vi "Yokogawa.vi"(0 "V/A ?":enum16{"DC V", "DC A"}(ring), 1 "Bias":enum16{"Low", "High"}(ring), 2 "Delay [ms]":u32=500, 3 "Messzeit [ms]":u32=5000, 4 "B-Feld":dbl, 5 "error in (no error)":errorcluster, 6 "Startwert":dbl=-5.0 min=-5.0 max=5.0 step=1.0, 7 "Stepsize":dbl=1.0 min=0.0, 8 "Endwert":dbl=5.0 min=-5.0 max=5.0 step=1.0) -> (15 "Ausgabe-Cluster":T1 {"Timestamp" format="%#_6f"}, 19 "error out":errorcluster)   [LabVIEW 2009]
uses:
  Instance           2 16Saved   Yokogawa .vi
panel:
  out "Done":bool
  out "Data":bool
  out "UI":dbl=12.99010000000002
  out "Modus":string="F1SA"
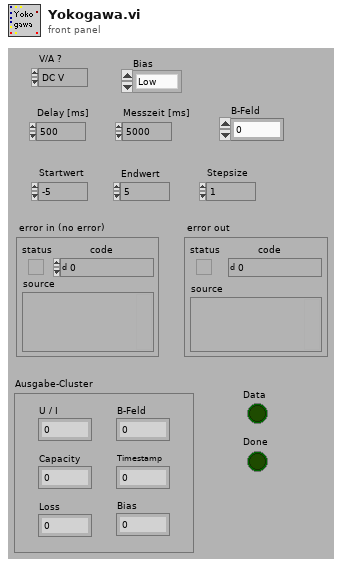
[diagram p1: front panel]
types:
  T1 = cluster{"U / I":dbl, "Capacity":dbl, "Loss":dbl, "B-Feld":dbl, "Timestamp":dbl, "Bias":u32}
  T2 = cluster{"UI":dbl, "capacitance":dbl, "loss":dbl, "B-Feld":dbl, dbl, "Bias":enum16{"Low", "High"}}
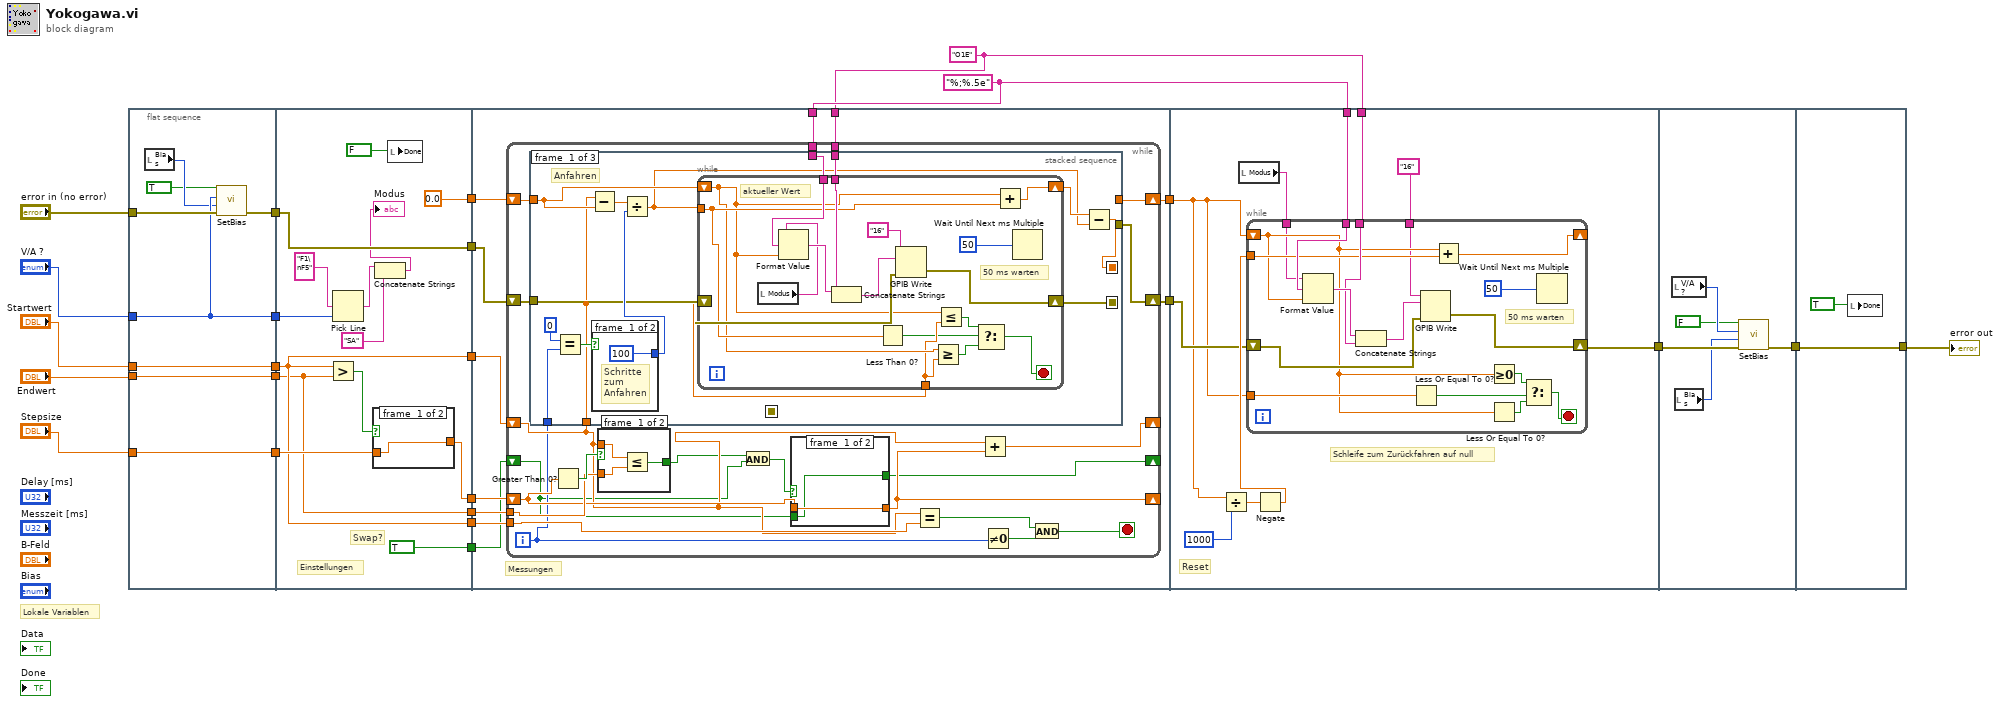
[diagram p0: block diagram]
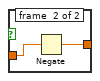
[diagram p2: hidden frame]
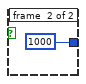
[diagram p3: hidden frame]
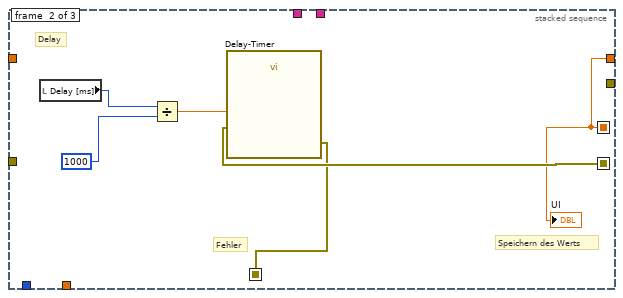
[diagram p4: hidden frame]
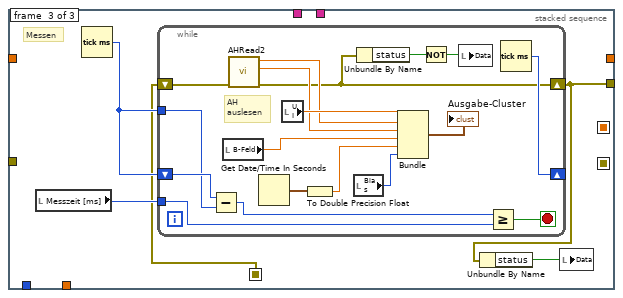
[diagram p5: hidden frame]
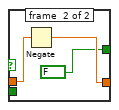
[diagram p6: hidden frame]
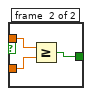
[diagram p7: hidden frame]
diagram:
  w9 = "O1E"
  w10 = "%;%.5e"
  # "Lokale Variablen"
  n1 = flat-sequence {
    tunnel: "Stepsize" -> [w30]
    tunnel: "Endwert" -> [w31]
    tunnel: "Startwert" -> [w32]
    tunnel: "V/A ?" -> [w27]
    tunnel: "error in (no error)" -> [w29]
    tunnel: [w28] -> w7
    tunnel: [w27] -> w6
    tunnel: [w32] -> w5
    tunnel: [w31] -> w4
    tunnel: [w30] -> w3
    tunnel: [w41] -> w19
    tunnel: [w42] -> w18
    tunnel: [w41] -> w17
    tunnel: [w40] -> w16
    tunnel: [0.0] -> w15
    tunnel: [w35] -> w14
    tunnel: [TRUE] -> w13
    tunnel: w7 -> [w35]
    tunnel: w6 -> [w45]
    tunnel: w5 -> [w41]
    tunnel: w4 -> [w40]
    tunnel: w3 -> [w43]
    tunnel: w19 -> [w60]
    tunnel: w18 -> [w58]
    tunnel: w17 -> [w59]
    tunnel: w16 -> [w57]
    tunnel: w15 -> [w56]
    tunnel: w10 -> [w55]
    tunnel: w9 -> [w54]
    tunnel: w14 -> [w53]
    tunnel: w13 -> [w51]
    tunnel: [w52] -> w12
    tunnel: [w50] -> w11
    tunnel: w12 -> [w159]
    tunnel: w11 -> [w157]
    tunnel: w10 -> [w161]
    tunnel: w9 -> [w160]
    tunnel: [w158] -> w2
    tunnel: w2 -> [w185]
    tunnel: [w186] -> w1
    tunnel: [w188] -> w8
    tunnel: w1 -> [w188]
    frame #0 {
      n2 = local read "Bias"() -> (w26:enum16{"Low", "High"})
      n3 = call "SetBias.vi"("error in (no error)"=w29, "Bias"=w26, "V/A ?"=w27, "On/Off"=TRUE) -> ("error out"=w28:errorcluster)  [unwired: 7 in]
    }
    frame #1 {
      # "Einstellungen"
      # "Swap?"
      n4 = Greater?(x=w41, y=w40) -> (0:w44:bool)
      n5 = Pick Line(multi-line string="F1\nF5", line index=w45) -> (output string=w38:string)  [unwired: 1 in]
      n6 = case shown="True" w44 {
        tunnel: w43 -> [w47 w49]
        tunnel: [w47 w48] -> w42
        frame #0 {
        }
        frame #1 {
          n7 = Negate(x=w49) -> (-x=w48:dbl)
        }
      }
      n8 = Concatenate Strings(w38, "SA") -> (→"Modus":string)
      n9 = local write "Done"(FALSE) -> ()
    }
    frame #2 {
      # "Messungen"
      n10 = while {
        shift-right: [w70] -> _
        shift-left: w60 -> [w72]
        tunnel: w59 -> [w81]
        shift-right: [w71] -> _
        shift-left: w58 -> [w78]
        tunnel: w57 -> [w79]
        shift-right: [w73] -> w50
        shift-left: w56 -> [w77]
        tunnel: w55 -> [w76]
        tunnel: w54 -> [w75]
        shift-right: [w69] -> w52
        shift-left: w53 -> [w74]
        shift-right: [w64] -> _
        shift-left: w51 -> [w62]
        i -> [w68]
        stop <- w65 stop-if-true
        n11 = stacked-sequence {
          seq-local: [w87 _ _] -> [_ w120 _]
          seq-local: [_ w119 _] -> [_ _ w123]
          seq-local: [w82 _ _] -> [_ w115 _]
          tunnel: w68 -> [w94 _ _]
          tunnel: w77 -> [w86 _ _]
          tunnel: w72 -> [w85 _ _]
          tunnel: w76 -> [w90 _ _]
          tunnel: w75 -> [w89 _ _]
          tunnel: w74 -> [w88 _ _]
          tunnel: [_ w115 _] -> w73
          tunnel: [_ _ w122] -> w69
          frame #0 {
            # "Anfahren"
            n12 = Equal?(x=0, y=w94) -> (x = y?=w95:bool)
            n13 = Subtract(x=w85, y=w86) -> (x-y=w92:dbl)
            n14 = case shown="True" w95 {
              tunnel: [100 1000] -> w91
              frame #0 {
                # "Schritte\nzum\nAnfahren"
              }
              frame #1 {
              }
            }
            n15 = Divide(x=w92, y=w91) -> (x/y=w83:dbl)
            n16 = while {
              shift-right: [w112] -> w84
              shift-left: w86 -> [w103]
              tunnel: w85 -> [w102]
              tunnel: w83 -> [w104]
              tunnel: w90 -> [w111]
              tunnel: w89 -> [w109]
              shift-right: [w106] -> w87
              shift-left: w88 -> [w107]
              stop <- w98 stop-if-true
              # "50 ms warten"
              # "aktueller Wert"
              n17 = local read "Modus"() -> (w96:string)
              n18 = Format Value(string ("")=w96, format string=w111, value (0)=w103) -> (output string=w110:string)
              n19 = Concatenate Strings(w110, w109) -> (w108:string)
              n20 = Less Than 0?(x=w104) -> (x < 0?=w101:bool)
              n21 = GPIB Write(0:"16", 1:w108, 3:w107) -> (6:w106:errorcluster)  [unwired: 2 in, 1 out]
              n22 = Greater Or Equal?(x=w103, y=w102) -> (x >= y?=w99:bool)
              n23 = Less Or Equal?(x=w103, y=w102) -> (x <= y?=w100:bool)
              n24 = Select(t=w100, s=w101, f=w99) -> (s? t:f=w98:bool)
              n25 = Add(x=w103, y=w104) -> (x+y=w112:dbl)
              n26 = Wait Until Next ms Multiple(millisecond multiple=50) -> ()  [unwired: 1 out]
            }
            n27 = Subtract(x=w84, y=w83) -> (x-y=w82:dbl)
          }
          frame #1 {
            # "Delay"
            # "Speichern des Werts"
            # "Fehler"
            n28 = local read "Delay [ms]"() -> (w116:u32)
            n29 = Divide(x=w116, y=u32 1000) -> (x/y=w117:dbl)
            n30 = call "Delay-Timer"("error in (no error)"=w120, "Delay Time (s)"=w117) -> ("error out"=w119:errorcluster)  [unwired: 9 in]
            "UI" <- w115
          }
          frame #2 {
            # "Messen"
            n31 = local read "Messzeit [ms]"() -> (w124:u32)
            n32 = Tick Count (ms)() -> (millisecond timer value=w125:u32)
            n33 = while {
              shift-right: [w143] -> _
              shift-left: w125 -> [w142]
              tunnel: w125 -> [w141]
              tunnel: w124 -> [w139]
              shift-right: [w127] -> w122
              shift-left: w123 -> [w137]
              stop <- w140 stop-if-true
              # "AH\nauslesen"
              n34 = Subtract(x=w142, y=w141) -> (x-y=w138:u32)
              n35 = local read "B-Feld"() -> (w131:dbl)
              n36 = call "AHRead2.vi"("error in (no error)"=w137) -> ("error out"=w127:errorcluster, "loss"=w132:dbl, "capacitance"=w133:dbl)  [unwired: 7 in, 1 out]
              n37 = Get Date/Time In Seconds() -> (seconds since 1Jan1904=w136:timestamp)
              n38 = local read "UI"() -> (w134:dbl)
              n39 = To Double Precision Float(number=w136) -> (double precision float=w130:dbl)
              n40 = local read "Bias"() -> (w129:enum16{"Low", "High"})
              n41 = Unbundle By Name(w127) -> ("status"=w128:bool)
              n42 = Bundle("UI"=w134, "capacitance"=w133, "loss"=w132, "B-Feld"=w131, w130, "Bias"=w129) -> (→"Ausgabe-Cluster":T2)  [unwired: 1 in]
              n43 = Not(x=w128) -> (.not. x?=w126:bool)
              n44 = local write "Data"(w126) -> ()
              n45 = Greater Or Equal?(x=w138, y=w139) -> (x >= y?=w140:bool)
              n46 = Tick Count (ms)() -> (millisecond timer value=w143:u32)
            }
            n47 = Unbundle By Name(w122) -> ("status"=w121:bool)
            n48 = local write "Data"(w121) -> ()
          }
        }
        n49 = Greater Than 0?(x=w78) -> (x > 0?=w80:bool)
        n50 = case shown="False" w80 {
          tunnel: w79 -> [w150 w153]
          tunnel: w72 -> [w151 w154]
          tunnel: [w149 w152] -> w63
          frame #0 {
            n51 = Less Or Equal?(x=w151, y=w150) -> (x <= y?=w149:bool)
          }
          frame #1 {
            n52 = Greater Or Equal?(x=w154, y=w153) -> (x >= y?=w152:bool)
          }
        }
        n53 = And(x=w63, y=w62) -> (x .and. y?=w61:bool)
        n54 = case shown="False" w61 {
          tunnel: w78 -> [w145 w148]
          tunnel: [w145 w147] -> w71
          tunnel: [w144 FALSE] -> w64
          tunnel: w62 -> [w144 _]
          frame #0 {
          }
          frame #1 {
            n55 = Negate(x=w148) -> (-x=w147:dbl)
          }
        }
        n56 = Equal?(x=w72, y=w81) -> (x = y?=w67:bool)
        n57 = Add(x=w72, y=w71) -> (x+y=w70:dbl)
        n58 = Not Equal To 0?(x=w68) -> (x != 0?=w66:bool)
        n59 = And(x=w67, y=w66) -> (x .and. y?=w65:bool)
      }
    }
    frame #3 {
      # "Schleife zum Zurückfahren auf null"
      # "Reset"
      n60 = Divide(x=w157, y=1000) -> (x/y=w163:dbl)
      n61 = local read "Modus"() -> (w155:string)
      n62 = Negate(x=w163) -> (-x=w162:dbl)
      n63 = while {
        shift-right: [w171] -> _
        shift-left: w157 -> [w168]
        tunnel: w162 -> [w175]
        tunnel: w161 -> [w181]
        tunnel: w160 -> [w179]
        shift-right: [w169] -> w158
        shift-left: w159 -> [w177]
        tunnel: w157 -> [w170]
        tunnel: "16" -> [w167]
        tunnel: w155 -> [w166]
        stop <- w165 stop-if-true
        # "50 ms warten"
        n64 = Format Value(string ("")=w166, format string=w181, value (0)=w168) -> (output string=w180:string)
        n65 = Concatenate Strings(w180, w179) -> (w178:string)
        n66 = Less Or Equal To 0?(x=w170) -> (x <= 0?=w174:bool)
        n67 = GPIB Write(0:w167, 1:w178, 3:w177) -> (6:w169:errorcluster)  [unwired: 2 in, 1 out]
        n68 = Add(x=w168, y=w175) -> (x+y=w171:dbl)
        n69 = Greater Or Equal To 0?(x=w168) -> (x >= 0?=w173:bool)
        n70 = Less Or Equal To 0?(x=w168) -> (x <= 0?=w172:bool)
        n71 = Select(t=w173, s=w174, f=w172) -> (s? t:f=w165:bool)
        n72 = Wait Until Next ms Multiple(millisecond multiple=50) -> ()  [unwired: 1 out]
      }
    }
    frame #4 {
      n73 = local read "V/A ?"() -> (w184:enum16{"DC V", "DC A"})
      n74 = local read "Bias"() -> (w183:enum16{"Low", "High"})
      n75 = call "SetBias.vi"("error in (no error)"=w185, "Bias"=w183, "V/A ?"=w184, "On/Off"=FALSE) -> ("error out"=w186:errorcluster)  [unwired: 7 in]
    }
    frame #5 {
      n76 = local write "Done"(TRUE) -> ()
    }
  }
  "error out" <- w8
